vi "Enqueue Enum (single).vi"(7 "Place at beginning (F)":bool, 8 "error in":errorcluster, 9 "Data":variant, 10 "State":i32, 11 "Queue In":refnum<queue>) -> (0 "error out":errorcluster, 3 "Queue Out":refnum<queue>)   [LabVIEW 2020, in "Enum Queue State Machine.lvlib"]
uses:
  Enum Queue State Machine.lvlib
  Controls/Enum Message.ctl
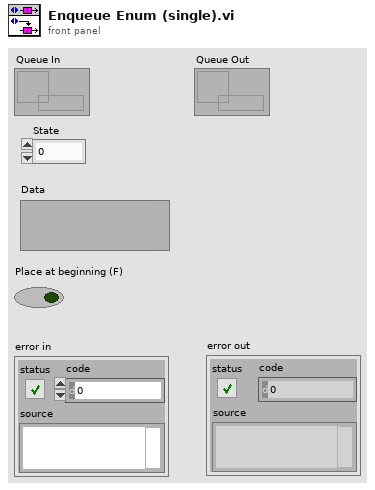
[diagram p1: front panel]
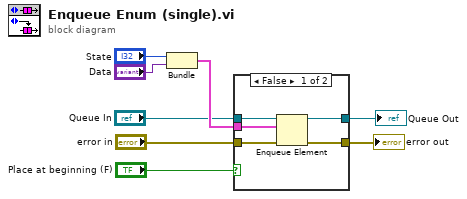
[diagram p0: block diagram]
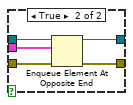
[diagram p2: hidden frame]
diagram:
  n1 = Bundle("State"="State", "Data"="Data") -> (w5:cluster{"State":i32, "Data":variant})  [unwired: 1 in]
  n2 = case shown="False" "Place at beginning (F)" {
    tunnel: "error in" -> [w11 w18]
    tunnel: [w10 w17] -> w7
    tunnel: "Queue In" -> [w13 w16]
    tunnel: [w12 w15] -> w1
    tunnel: w5 -> [w9 w14]
    frame False {
      n3 = Enqueue Element(queue=w13, element=w9, error in (no error)=w11) -> (queue out=w12:refnum<queue>, error out=w10:errorcluster)  [unwired: 1 in, 1 out]
    }
    frame True {
      n4 = Enqueue Element At Opposite End(queue=w16, element=w14, error in (no error)=w18) -> (queue out=w15:refnum<queue>, error out=w17:errorcluster)  [unwired: 1 in, 1 out]
    }
  }
  "error out" <- w7
  "Queue Out" <- w1
